vi "test2.vi"() -> ()   [LabVIEW 2010]
panel:
  out "DeviceOpen":bool
  in  "stop":bool
  out "Response":string
  in  "Command":string
  in  "deviceKey IN":string
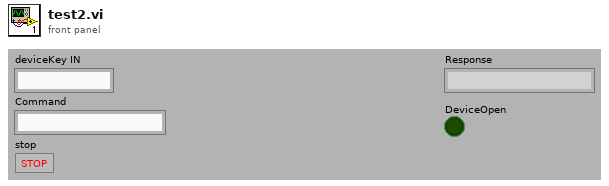
[diagram p1: front panel]
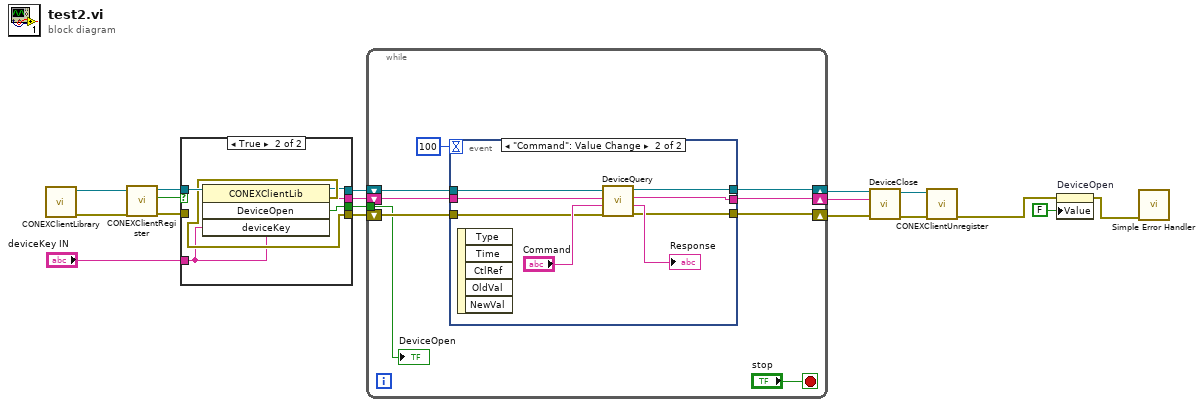
[diagram p0: block diagram]
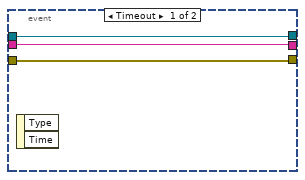
[diagram p2: hidden frame]
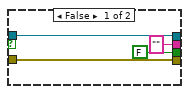
[diagram p3: hidden frame]
diagram:
  n1 = call <userlib>:"CONEXClientLibrary.vi"() -> ("CONEX Client LIB ref"=w18:refnum<k24>, "Error OUT"=w17:errorcluster)  [unwired: 4 in]
  n2 = call <userlib>:"CONEXClientRegister.vi"("Error IN"=w17, "CONEX Client Lib Ref"=w18) -> ("Error OUT"=w15:errorcluster, "Connect?"=w14:bool, "CONEX Client Ref"=w16:refnum<k24>)  [unwired: 7 in]
  n3 = case shown="True" w14 {
    tunnel: w16 -> [w22 w27]
    tunnel: w15 -> [w21 _]
    tunnel: "deviceKey IN" -> [_ w24]
    tunnel: [w22 w23] -> w12
    tunnel: ["" ("deviceKey OUT") w24] -> w11
    tunnel: [FALSE ("DeviceOpen") w26] -> w10
    tunnel: [w21 w25] -> w9
    frame False {
    }
    frame True {
      n4 = invoke class="CONEXClientLib" method="DeviceOpen"(reference=w27, "deviceKey"=w24) -> (reference out=w23:refnum<k24>, error out=w25:errorcluster, "DeviceOpen"=w26:bool)  [unwired: 2 in, 1 out]
    }
  }
  n5 = while {
    tunnel: w10 -> [w28]
    shift-right: [w30] -> w7
    shift-left: w9 -> [w34]
    shift-right: [w32] -> w8
    shift-left: w12 -> [w36]
    shift-right: [w31] -> w6
    shift-left: w11 -> [w35]
    stop <- "stop" stop-if-true
    n6 = event shown="[1] \"Command\": Value Change" {
      selector: _ -> [_ _]
      dyn-events: _ -> [_ _]
      timeout: 100 -> [_ _]
      tunnel: w36 -> [w39 w45]
      tunnel: w35 -> [w38 w44]
      tunnel: w34 -> [w37 w43]
      tunnel: [w39 w42] -> w32
      tunnel: [w38 w41] -> w31
      tunnel: [w37 w40] -> w30
      event Timeout {
        n7 = event-data() -> ()  [unwired: 1 in, 2 out]
      }
      event "Command": Value Change {
        n8 = event-data() -> ()  [unwired: 1 in, 5 out]
        n9 = call <userlib>:"DeviceQuery.vi"("Error IN"=w43, "Command"="Command", "deviceKey IN"=w44, "CONEX Client Ref IN"=w45) -> ("Error OUT"=w40:errorcluster, "Response"=→"Response":string, "deviceKey OUT"=w41:string, "CONEX Client Ref OUT"=w42:refnum<k24>)  [unwired: 4 in]
      }
    }
    "DeviceOpen" <- w28
  }
  n10 = call <userlib>:"DeviceClose.vi"("Error IN"=w7, "deviceKey IN"=w6, "CONEX Client Ref IN"=w8) -> ("Error OUT"=w5:errorcluster, "CONEX Client Ref OUT"=w4:refnum<k24>)  [unwired: 6 in, 1 out]
  n11 = call <userlib>:"CONEXClientUnregister.vi"("Error IN"=w5, "CONEX Client Ref IN"=w4) -> ("Error OUT"=w2:errorcluster)  [unwired: 8 in, 1 out]
  n12 = property on="DeviceOpen" class="Bool (strict)"(error in=w2, "Value"=FALSE ("DeviceOpen")) -> (error out=w1:errorcluster)  [unwired: 1 in, 1 out]
  n13 = call <vilib>:"Simple Error Handler.vi"("error in (no error)"=w1) -> ()  [unwired: 4 in, 5 out]
